vi "GetDataSubVi.vi"(10 "Expt name":string="Staging", 11 "Stop 2":refnum<vi>) -> ()   [LabVIEW 2020]
uses:
  Shared/Device Driver/GUIDeviceInfo_TypDEf.ctl
  Shared/MySQL/Preset Query Enum.ctl
  Shared/GUI_Template/GUI_master/tcp new data cluster.ctl
  Controls/diagnosticQuee.ctl
  <vilib>/Analysis/1siggen.llb/Ramp Pattern by Samples.vi
  <vilib>/Analysis/NI_AALBase.lvlib
panel:
  out "timing Graph":cluster{i32[], "Ramp Pattern":dbl[]}(graph)
  in  "Stop":bool=TRUE
  in  "GUIDeviceInfo":T1
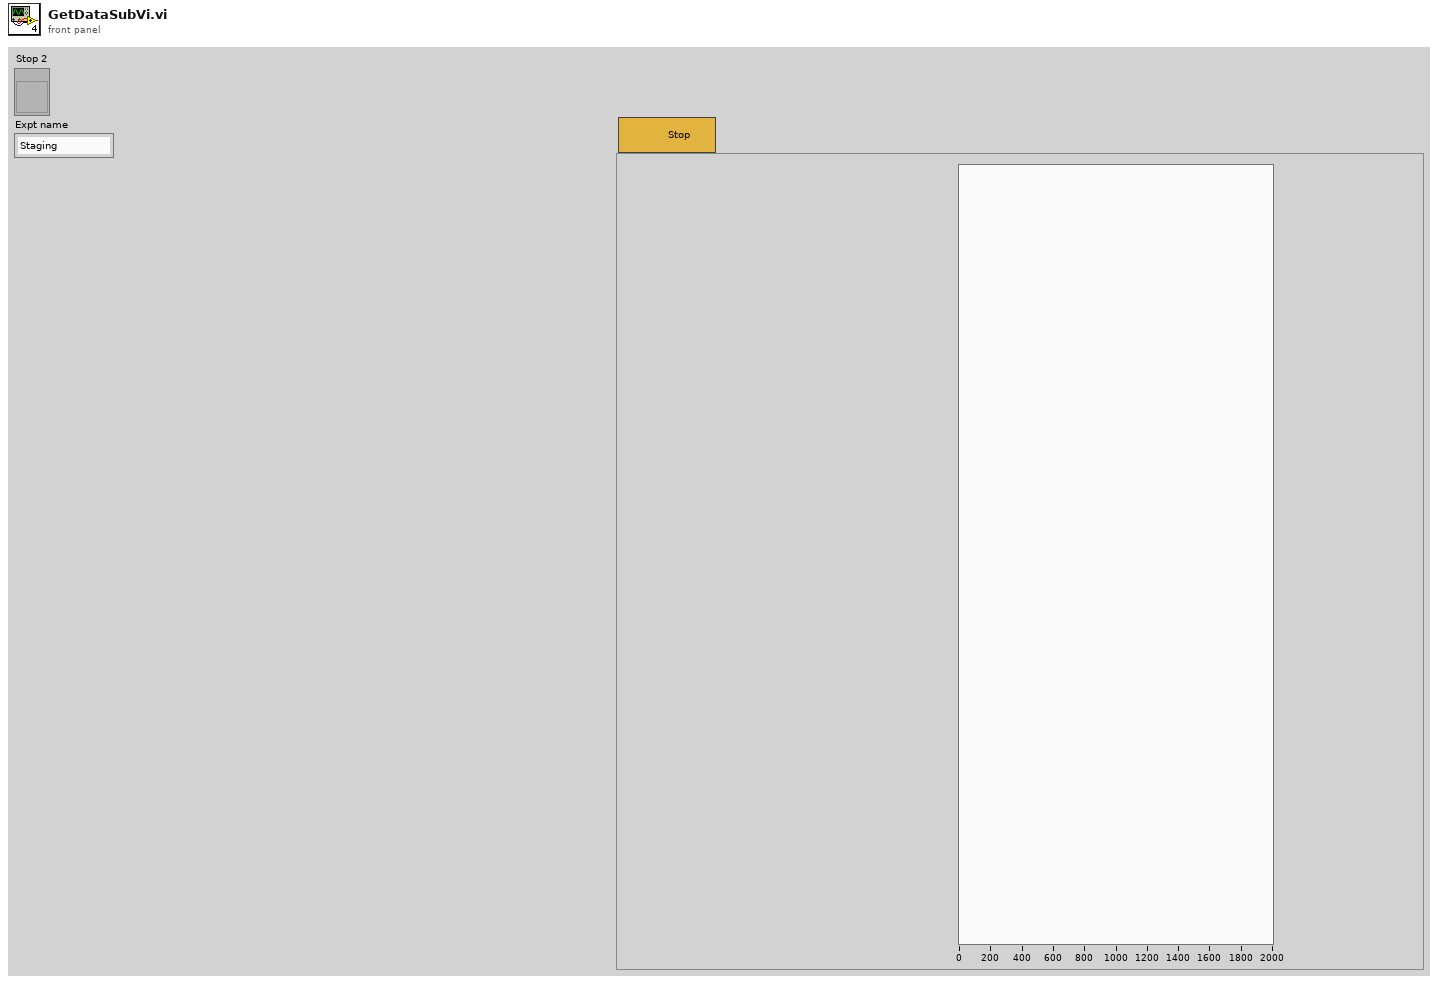
[diagram p1: front panel]
types:
  T1 = typedef "GUIDeviceInfo_TypDEf.ctl" = cluster{"device space variable array":string[], "subscribe messages for process vis":string[], "variable list (ordered as controls)":string[], "Device Controles":refnum<vi>[], "IP addresses":string[], "Ports":string[], "Devices (groups)":string[], "Channel Enum Ref":refnum<vi>[], "Enable Subscribe":string[], "Devices names":string[], "variable limits":string[][], "GUI Controls ":refnum<vi>[], "stop ref":refnum<vi>, "Caller VI ref":refnum<vi>, "UDP error message":refnum<vi>, "refresh button":refnum<vi>}
  T2 = typedef "Preset Query Enum.ctl" = enum16{"Get Locations", "Get all IPs and MACs", "Get classes", "Get expt variables to set at scanstart for particular device", "Get expt devices and variables with start values", "Get expt devices and variables (with data to get)", "Get expt devices with data to get", "Get Expt devices and GUIs", "Get all devices basic properties", "Get Virtual Devices Core Info", "Get Expt names", "Get experiment basic properties", "Get experiment alarm variables", "Get MC Ports", "Get device network comm port", "Get devicetype lvclass path", "Get basic device properties", "Get Init Order", "Get all setable variables of a device", "Get device variable aliases", "Get force values of all settable variables", "Get all variables of a devicetype", "Get all variables of a device", "Get plotter details", "Get Saved Scans", "Get Scan Info", "GetGeneralGUIs", "Get expt for plotter", "Get plotter IDs from expt", "Get all devices", "Get all Virtual Devices", "Get all aliases", "Get variable and device info for Virtual Device", "GetItemLocatorIP", "Get IPs for GUIs", "Get DeviceType from Device", "GetLocalPortRange", "GetDevicePresetVariables", "Get Device Configuration", "GetAllPresetNames", "GetAllConfigurationNames", "GetPresetDeviceNames", "GetDeviceAliases", "GetDevicesOfClass"}
  T3 = typedef "diagnosticQuee.ctl" = cluster{"device":string[], "error":string[], "ststus":string[], "timing graph":cluster{u32[], "Ramp Pattern":dbl[]}, "error boolean":bool[], "error history":string[]}
  T4 = typedef "tcp new data cluster.ctl" = cluster{"EventEnum":enum16{"new data", "connection status update"}, "Device name":string}
  T5 = typedef "QueueCluster.ctl" = cluster{"UDP":refnum<queue>, "Data":refnum<queue>, "Stop":refnum<queue>, "Control":refnum<queue>, "tcp data event":refnum<user-event>, "Event Registration Refnum":refnum<event-registration>}
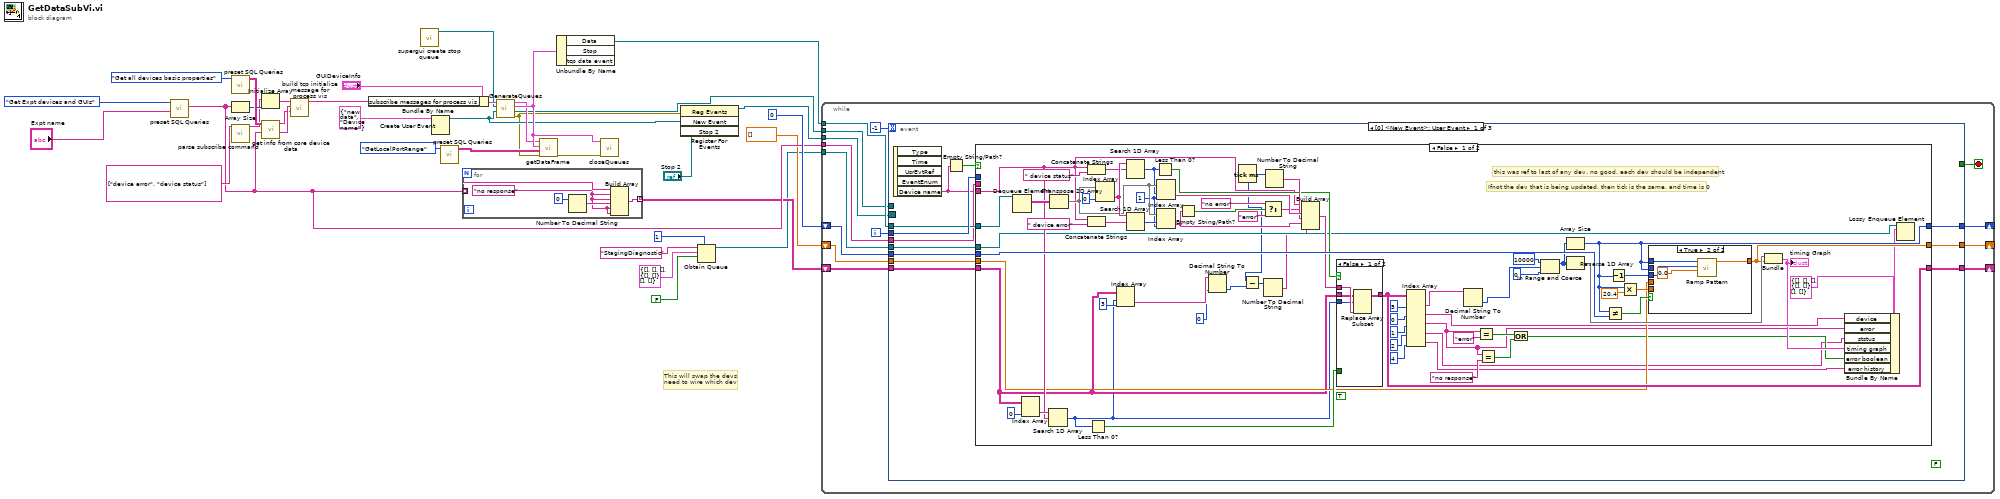
[diagram p0: block diagram]
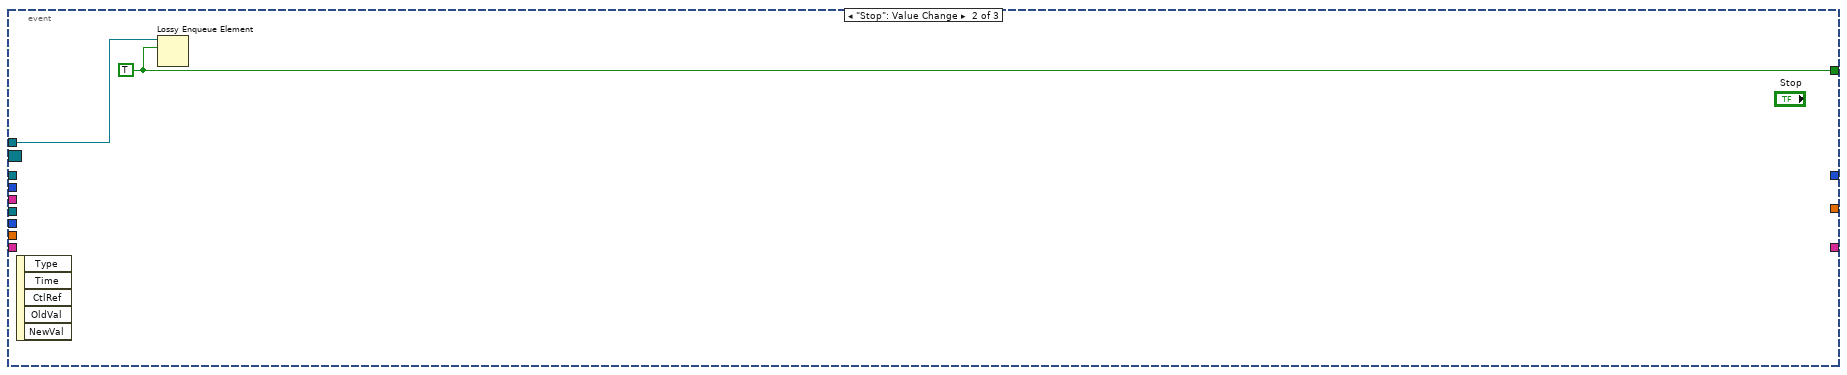
[diagram p5: hidden frame]
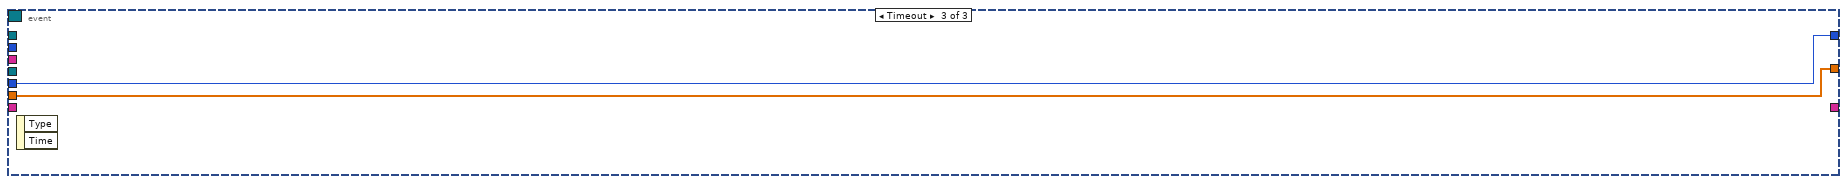
[diagram p6: hidden frame]
diagram:
  # "This will swap the devs\nneed to wire which dev"
  n1 = call "preset SQL Queries.vi"("Expt name / MCIP/ Variable/Preset Name"="Expt name", "Preset Query"=Preset_Query_Enum."Get Expt devices and GUIs") -> ("1st column 1st data"=w15:string[])  [unwired: 7 in, 2 out]
  n2 = call "preset SQL Queries.vi"("Preset Query"=Preset_Query_Enum."Get all devices basic properties") -> ("data"=w32:string[][])  [unwired: 8 in, 2 out]
  n3 = Array Size(array=w15) -> (size(s)=w23:i32)
  n4 = call "parse subscribe command.vi"("variable names"=string[] ["device error", "device status"]) -> ("Subscribe command"=w22:string)  [unwired: 6 in]
  n5 = Initialize Array(w22, w23) -> (w21:string[])
  n6 = call "get info from core device data.vi"("devices to get data from"=w15, "All Devices Core Info"=w32) -> ("Ports"=w31:string[], "IP Addresses"=w30:string[])  [unwired: 1 in, 3 out]
  n7 = call "build tcp initialize message for process vis.vi"("IP Addresses"=w30, "Ports"=w31, "Subscribe commands"=w21) -> ("subscribe messages\nfor process vis"=w29:string[])  [unwired: 8 in]
  n8 = Bundle By Name(cluster="GUIDeviceInfo", "subscribe messages for process vis"=w29) -> (w26:T1)
  n9 = call "supergui create stop queue.vi"() -> ("STOP Queue out"=w4:refnum<queue>)  [unwired: 11 in]
  n10 = Create User Event(user event datatype=T4 {"EventEnum"=enum."new data", "Device name"="Device name"} ("New Event")) -> (user event=w2:refnum<user-event>)  [unwired: 1 in, 1 out]
  n11 = call "preset SQL Queries.vi"("Preset Query"=Preset_Query_Enum."GetLocalPortRange") -> ("data"=w5:string[][])  [unwired: 8 in, 2 out]
  n12 = for {
    tunnel: w15 -> [w40] mode=indexing
    tunnel: [w37] -> w14 mode=indexing
    w36 = "no response" ("element")
    n13 = Number To Decimal String(number=0) -> (decimal integer string=w38:string)  [unwired: 1 in]
    n14 = Build Array(w40, w36, w36, w38, w36, w36) -> (w37:string[])
  }
  n15 = call "GenerateQueues.vi"("User Event in"=w2, "STOP Queue in"=w4, "GUIDeviceInfo"=w26) -> ("error out"=w1:errorcluster, "Stop Queue out"=w3:refnum<queue>, "Queue Cluster"=w34:T5, "GUIDeviceInfoout"=w25:T1)  [unwired: 4 in, 1 out]
  n16 = call "getDataFrame.vi"("error in (no error)"=w1, "Ports"=w5, "Queue Cluster"=w34, "GUIDeviceInfo"=w25) -> ("error out"=w35:errorcluster)  [unwired: 7 in]
  n17 = Unbundle By Name(w34) -> ("Data"=w20:refnum<queue>)  [unwired: 2 out]
  n18 = call "closeQueues.vi"("error in (no error)"=w35, "Queue Cluster"=w34) -> ()  [unwired: 9 in, 1 out]
  n19 = register-events(error in=w1, w2, "Stop 2") -> (reference out=w28:refnum<event-registration>)  [unwired: 1 in, 1 out]
  n20 = Obtain Queue(max queue size (-1, unlimited)=1, name (unnamed)="StagingDiagnostic", element data type=T3 {"device"=[], "error"=[], "ststus"=[], "timing graph"={[], "Ramp Pattern"=[]}, "error boolean"=[], "error history"=[]} ("output cluster"), create if not found? (T)=FALSE) -> (queue out=w9:refnum<queue>)  [unwired: 1 in, 2 out]
  n21 = while {
    tunnel: w3 -> [w43]
    tunnel: w28 -> [w46]
    tunnel: w20 -> [w52]
    shift-right: [w50] -> _
    shift-left: w14 -> [w51]
    tunnel: w15 -> [w49]
    shift-right: [w48] -> _
    shift-left: u32 0 ("Number of Rows") -> [w47]
    shift-right: [w45] -> _
    shift-left: dbl[] [] ("Ramp Pattern") -> [w44]
    tunnel: w9 -> [w41]
    i -> [w53]
    stop <- w42 stop-if-true
    n22 = event shown="[0] <New Event>: User Event" {
      selector: w46 -> [_ _ _]
      dyn-events: _ -> [_ _ _]
      timeout: -1 -> [_ _ _]
      tunnel: w53 -> [w66 _ _]
      tunnel: w52 -> [w65 _ _]
      tunnel: w51 -> [w64 _ _]
      tunnel: [w63 _ _] -> w50
      tunnel: w49 -> [w60 _ _]
      tunnel: [w62 _ w149] -> w48
      tunnel: w47 -> [w61 _ w149]
      tunnel: [w57 _ w150] -> w45
      tunnel: w44 -> [w56 _ w150]
      tunnel: [_ w147 _] -> w42
      tunnel: w43 -> [_ w148 _]
      tunnel: w41 -> [w55 _ _]
      event User Event {
        (unwired) FALSE
        n23 = event-data() -> ("Device name"=w58:string)  [unwired: 1 in, 4 out]
        n24 = Empty String/Path?(string/path=w58) -> (empty?=w59:bool)
        n25 = case shown="False" w59 {
          tunnel: w66 -> [_ _]
          tunnel: w65 -> [w130 _]
          tunnel: w64 -> [w76 w146]
          tunnel: [w125 w146] -> w63
          tunnel: w60 -> [_ _]
          tunnel: [w91 w145] -> w62
          tunnel: w61 -> [w122 w145]
          tunnel: w58 -> [w92 _]
          tunnel: [w89 w144] -> w57
          tunnel: w56 -> [w88 w144]
          tunnel: w55 -> [w84 _]
          frame False {
            w103 = 1 ("disabled index (col)")
            (unwired) TRUE
            # "Ifnot the dev that is being updated, then tick is the same, and time is 0"
            # "this was ref to last of any dev. no good. each dev should be independent"
            n26 = Dequeue Element(queue=w130) -> (element=w131:string[][])  [unwired: 2 in, 3 out]
            n27 = Index Array(array=w76, index (col)=0 ("disabled index (col)")) -> (element=w132:string[])  [unwired: 1 in]
            n28 = Search 1D Array(1D array=w132, element=w92) -> (index of element=w74:i32)  [unwired: 1 in]
            n29 = Transpose 2D Array(2D array=w131) -> (transposed array=w104:string[][])
            n30 = Concatenate Strings(w92, " device status" ("String")) -> (w105:string)
            n31 = Concatenate Strings(w92, " device error" ("String")) -> (w111:string)
            n32 = Less Than 0?(x=w74) -> (x < 0?=w109:bool)
            n33 = Index Array(array=w104, index (col)=0 ("index (row)")) -> (element=w106:string[])  [unwired: 1 in]
            n34 = Index Array(array=w76, index (row)=w74, index (col)=3 ("disabled index (col)")) -> (element=w75:string)
            n35 = Search 1D Array(1D array=w106, element=w105) -> (index of element=w94:i32)  [unwired: 1 in]
            n36 = Search 1D Array(1D array=w106, element=w111) -> (index of element=w110:i32)  [unwired: 1 in]
            n37 = Less Than 0?(x=w94) -> (x < 0?=w93:bool)
            n38 = Index Array(array=w104, index (row)=w94, index (col)=w103) -> (element=w102:string)
            n39 = Index Array(array=w104, index (row)=w110, index (col)=w103) -> (element=w95:string)
            n40 = Empty String/Path?(string/path=w95) -> (empty?=w99:bool)
            n41 = Decimal String To Number(string=w75, default (0L)=u32 0 ("default (0 I32)")) -> (number=w72:u32)  [unwired: 1 in, 1 out]
            n42 = Tick Count (ms)() -> (millisecond timer value=w73:u32)
            n43 = Subtract(x=w73, y=w72) -> (x-y=w71:u32)
            n44 = Select(t="no error", s=w99, f="error") -> (s? t:f=w97:string)
            n45 = Number To Decimal String(number=w71) -> (decimal integer string=w70:string)  [unwired: 1 in]
            n46 = Number To Decimal String(number=w73) -> (decimal integer string=w100:string)  [unwired: 1 in]
            n47 = Build Array(w92, w97, w102, w100, w95, w70) -> (w101:string[])
            n48 = case shown="False" w93 {
              tunnel: w109 -> [_ _]
              tunnel: w76 -> [w135 w138]
              tunnel: w74 -> [w134 _]
              tunnel: w101 -> [w137 _]
              tunnel: [w136 w138] -> w125
              frame False {
                n49 = Replace Array Subset(array=w135, new element=w137, index (row)=w134) -> (w136:string[][])  [unwired: 1 in]
              }
              frame True {
              }
            }
            n50 = Index Array(array=w125, index (col) #1=5 ("disabled index (col)"), index (col) #2=0 ("index (col)"), index (col) #3=1 ("index (col)"), index (col) #4=2 ("index (col)"), index (col) #5=4 ("index (col)")) -> (element #1=w69:string[], element #2=w87:string[], element #3=w78:string[], element #4=w79:string[], element #5=w80:string[])  [unwired: 5 in]
            n51 = Decimal String To Number(string=w69) -> (number=w68:i32[])  [unwired: 2 in, 1 out]
            n52 = Equal?(x=w78, y="error") -> (x = y?=w115:bool[])
            n53 = Equal?(x=w78, y="no response" ("element")) -> (x = y?=w114:bool[])
            n54 = Or(x=w115, y=w114) -> (x .or. y?=w82:bool[])
            n55 = In Range and Coerce(upper limit=10000, x=w68, lower limit=0) -> (coerced(x)=w117:i32[])  [unwired: 1 out]
            n56 = Array Size(array=w117) -> (size(s)=w91:i32)
            n57 = Reverse 1D Array(array=w117) -> (reversed array=w127:i32[])
            n58 = Not Equal?(x=w91, y=w122) -> (x != y?=w121:bool)
            n59 = Decrement(x=w91) -> (x-1=w90:i32)
            n60 = Multiply(x=w91, y=20.4) -> (x*y=w123:dbl)
            n61 = case shown="True" w121 {
              tunnel: w91 -> [_ _]
              tunnel: w123 -> [_ _]
              tunnel: w91 -> [_ w143]
              tunnel: w90 -> [_ w142]
              tunnel: [w139 w140] -> w89
              tunnel: w88 -> [w139 _]
              frame False {
              }
              frame True {
                n62 = call-poly <vilib>:"Ramp Pattern.vi"("start"=0.0, "end"=w142, "samples"=w143) -> ("Ramp Pattern"=w140:dbl[])  [unwired: 7 in, 1 out]
              }
            }
            n63 = Bundle(w127, "Ramp Pattern"=w89) -> (w86:cluster{i32[], "Ramp Pattern":dbl[]})  [unwired: 1 in]
            "timing Graph" <- w86
            n64 = Bundle By Name(cluster=T3 {"device"=[], "error"=[], "ststus"=[], "timing graph"={[], "Ramp Pattern"=[]}, "error boolean"=[], "error history"=[]} ("output cluster"), "device"=w87, "error"=w78, "ststus"=w79, "timing graph"=w86, "error boolean"=w82, "error history"=w80) -> (w85:T3)
            n65 = Lossy Enqueue Element(queue=w84, element=w85) -> ()  [unwired: 1 in, 4 out]
          }
          frame True {
          }
        }
      }
      event "Stop": Value Change {
        w147 = TRUE
        n66 = event-data() -> ()  [unwired: 1 in, 5 out]
        n67 = Lossy Enqueue Element(queue=w148, element=w147) -> ()  [unwired: 1 in, 4 out]
      }
      event Timeout {
        n68 = event-data() -> ()  [unwired: 1 in, 2 out]
      }
    }
  }
